vi "Write Error.vi"(8 "error in (no error)":errorcluster, 10 "Error":sgl, 11 "Stability Data in":refnum<class "Stability Data.lvclass">) -> (0 "error out":errorcluster, 3 "Stability Data out":refnum<class "Stability Data.lvclass">)   [LabVIEW 2015, in "Stability Data.lvclass"]
uses:
  Stability Data.lvclass
  Stability Data.lvclass/Stability Data.ctl
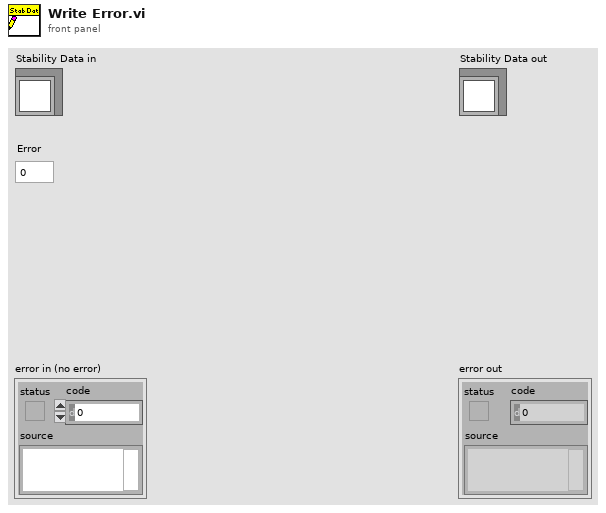
[diagram p1: front panel]
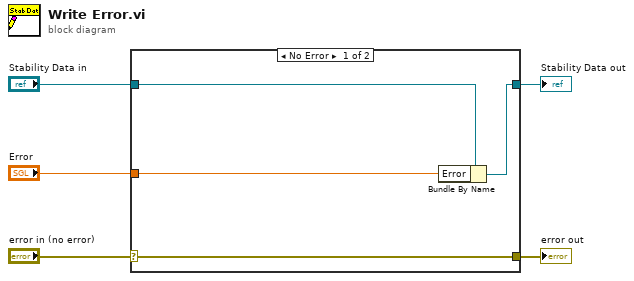
[diagram p0: block diagram]
diagram:
  n1 = case shown="No Error" "error in (no error)" {
    selector: "error in (no error)" -> [w9 w10]
    tunnel: [w9 w10] -> w4
    tunnel: [w7 w11] -> w2
    tunnel: "Stability Data in" -> [w8 w11]
    tunnel: "Error" -> [w6 _]
    frame No Error {
      n2 = Bundle By Name(cluster=w8, "Error"=w6) -> (w7:refnum<class "Stability Data.lvclass">)
    }
    frame Error {
    }
  }
  "error out" <- w4
  "Stability Data out" <- w2
